vi "Read Configuration Data.vi"(8 "error in":errorcluster) -> (0 "error out":errorcluster, 3 "MHL Configuration":T1)   [LabVIEW 2014]
uses:
  controls/MHL Configuration.ctl
  Boiler System Globals.vi
  <vilib>/Utility/config.llb/NI_LVConfig.lvlib
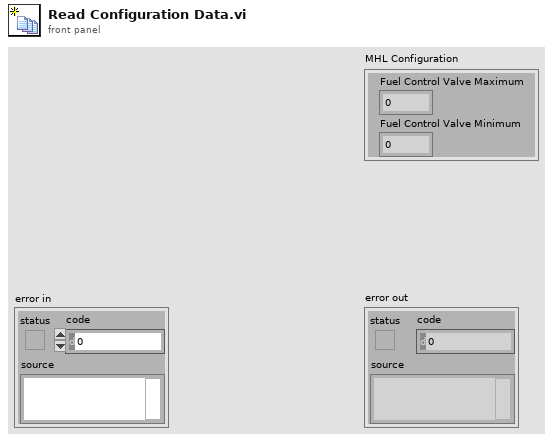
[diagram p1: front panel]
types:
  T1 = typedef "MHL Configuration.ctl" = cluster{"Fuel Control Valve Maximum":dbl, "Fuel Control Valve Minimum":dbl}
  T2 = enum32{"invalid app kind", "Development System", "Run Time System", "Student Edition", "Embedded LabVIEW", "Evaluation", "Custom"}
  T3 = typedef "NI_LVConfig.lvlib/Config Data RefNum.ctl" = refnum<k1>
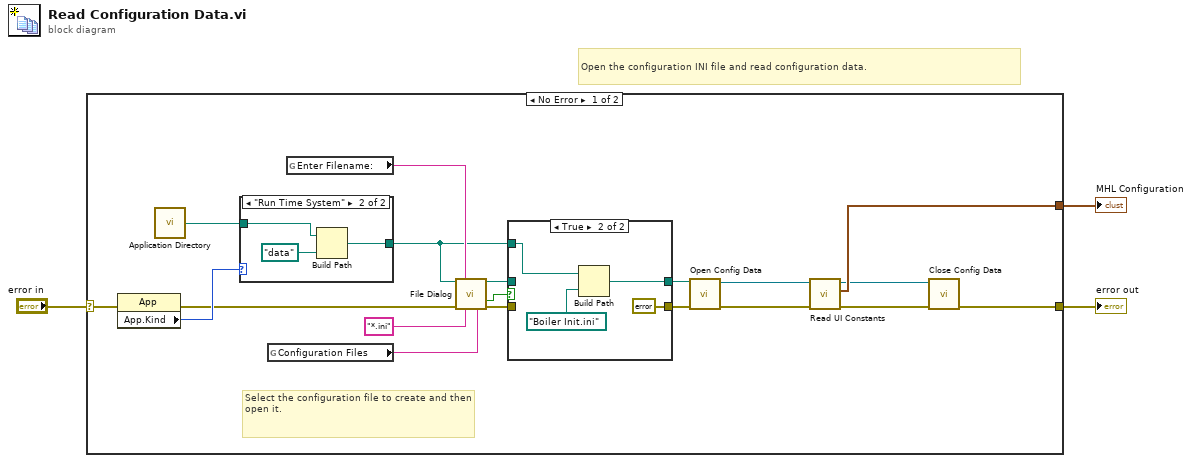
[diagram p0: block diagram]
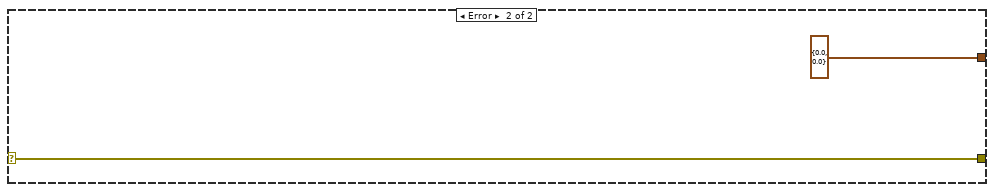
[diagram p4: hidden frame]
diagram:
  # "Open the configuration INI file and read configuration data."
  n1 = case shown="No Error" "error in" {
    selector: "error in" -> [w11 w34]
    tunnel: [w17 w34] -> w3
    tunnel: [w15 T1 {"Fuel Control Valve Maximum"=0.0, "Fuel Control Valve Minimum"=0.0} ("MHL Configuration")] -> w2
    frame No Error {
      # "Select the configuration file to create and then open it."
      n2 = property class="App"(error in=w11) -> (error out=w10:errorcluster, "App.Kind"=w13:T2)  [unwired: 1 in, 1 out]
      n3 = call <vilib>:"Application Directory.vi"() -> ("Application Directory"=w12:path)
      n4 = case shown="\"Run Time System\"" w13 {
        tunnel: w12 -> [w29 w32]
        tunnel: [w29 w30] -> w4
        frame Default {
        }
        frame "Run Time System" {
          n5 = Build Path(base path=w32, name or relative path=path "data") -> (appended path=w30:path)
        }
      }
      n6 = global read "Boiler System Globals.vi" "Configuration Files"() -> (w20:string)
      n7 = global read "Boiler System Globals.vi" "Enter Filename:"() -> (w22:string)
      n8 = call "File Dialog"("start path"=w4, "prompt"=w22, "error in"=w10, "pattern (all files)"="*.ini", "pattern label"=w20) -> ("selected path"=w7:path, "cancelled"=w9:bool, "error out"=w8:errorcluster)  [unwired: 7 in, 1 out]
      n9 = case shown="True" w9 {
        tunnel: w8 -> [w24 _]
        tunnel: w7 -> [w23 _]
        tunnel: [w24 errorcluster {"status"=FALSE, "code"=0, "source"=""} ("error out")] -> w6
        tunnel: [w23 w27] -> w5
        tunnel: w4 -> [_ w28]
        frame False {
        }
        frame True {
          n10 = Build Path(base path=w28, name or relative path=path "Boiler Init.ini") -> (appended path=w27:path)
        }
      }
      n11 = call <vilib>:"Open Config Data.vi"("error in (no error)"=w6, "configuration file path"=w5) -> ("error out"=w18:errorcluster, "refnum"=w19:T3)  [unwired: 1 in, 7 out]
      n12 = call "Read UI Constants.vi"("error in"=w18, "CFG File Refnum in"=w19) -> ("error out"=w16:errorcluster, "MHL Configuration"=w15:T1, "CFG File Refnum out"=w14:T3)  [unwired: 7 in]
      n13 = call <vilib>:"Close Config Data.vi"("error in (no error)"=w16, "refnum"=w14) -> ("error out"=w17:errorcluster)  [unwired: 1 in, 8 out]
    }
    frame Error {
    }
  }
  "error out" <- w3
  "MHL Configuration" <- w2
